vi "Set Module Configuration Revision from Identifier.vi"(8 "error in (no error)":errorcluster, 9 "Revision":u32, 10 "Module identifier":string, 11 "Routing and Faulting Ref in":T1 format="%.0x") -> (0 "error out":errorcluster, 3 "Routing and Faulting Ref out":T1 format="%.0x")   [LabVIEW 2017, in "Routing and Faulting Scripting.lvlib"]
uses:
  Routing and Faulting Scripting.lvlib
  <vilib>/NI Veristand/Custom Device API/Custom Device Item Ref.ctl
  NationalInstruments.VeriStand.SystemStorage
  <vilib>/NI Veristand/Custom Device API/Custom Device API.lvlib
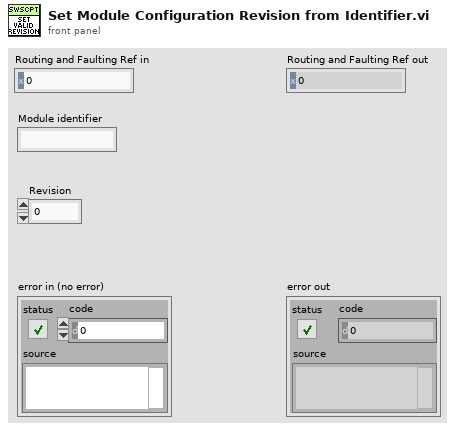
[diagram p1: front panel]
types:
  T1 = typedef "Custom Device API.lvlib/Custom Device Item Ref.ctl" = u64
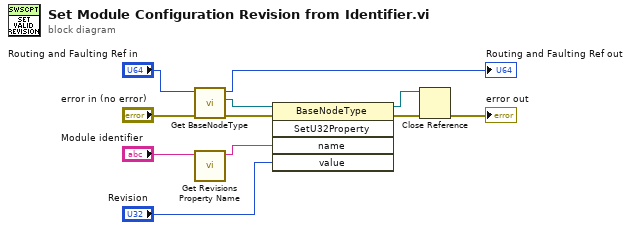
[diagram p0: block diagram]
diagram:
  n1 = call "Get BaseNodeType.vi"("error in (no error)"="error in (no error)", "Item Ref in"="Routing and Faulting Ref in") -> ("error out"=w10:errorcluster, "BaseNodeType"=w7:refnum<k24>, "Item Ref out"=→"Routing and Faulting Ref out":T1)  [unwired: 7 in]
  n2 = call "Get Revisions Property Name.vi"("Module ID"="Module identifier") -> ("Module Property Name"=w5:string)  [unwired: 10 in]
  n3 = invoke class="BaseNodeType" method="SetU32Property"(reference=w7, error in=w10, "name"=w5, "value"="Revision") -> (reference out=w3:refnum<k24>, error out=w4:errorcluster)  [unwired: 1 in, 3 out]
  n4 = Close Reference(reference=w3, error in (no error)=w4) -> (error out=→"error out":errorcluster)
